vi "Phase and Amplitude Matching 2012NIVerified.vi"() -> ()   [LabVIEW 2018]
doc: "This example executes phase and/or amplitude alignment for two waveforms of the same frequency"
uses:
  <vilib>/measure/matone.llb/Extract Single Tone Information 1 Chan.vi
  <vilib>/measure/maresamp.llb/Align two Waveforms (continuous).vi
  <vilib>/measure/NI_MAPro.lvlib
  <vilib>/measure/NI_MABase.lvlib
panel:
  out "Processed Waveforms":waveform(dbl)[](graph)
  in  "Enable Phase Match?":bool=TRUE
  in  "Enable Amplitude Match?":bool=TRUE
  in  "Sampling Info A":cluster{"Fs":dbl, "#s":dbl}={"Fs"=1000.0, "#s"=1000.0}
  in  "Phase A":dbl=45.0
  in  "Amplitude A":dbl=5.0
  in  "Sampling Info B":cluster{"Fs":dbl, "#s":dbl}={"Fs"=1000.0, "#s"=1000.0}
  in  "Phase B":dbl=180.0
  in  "Amplitude B":dbl=1.0
  in  "Waveform Frequency":dbl=10.0
  out "Original Waveforms":waveform(dbl)[](graph)
  # "Overview: This example executes phase and/or amplitude alignment for two waveforms of the same frequency.\nRequirements: LabVIEW 2012 or compatible\nInstructions:\n1Run VI"
  # "Waveform A Properties"
  # "Waveform B Properties"
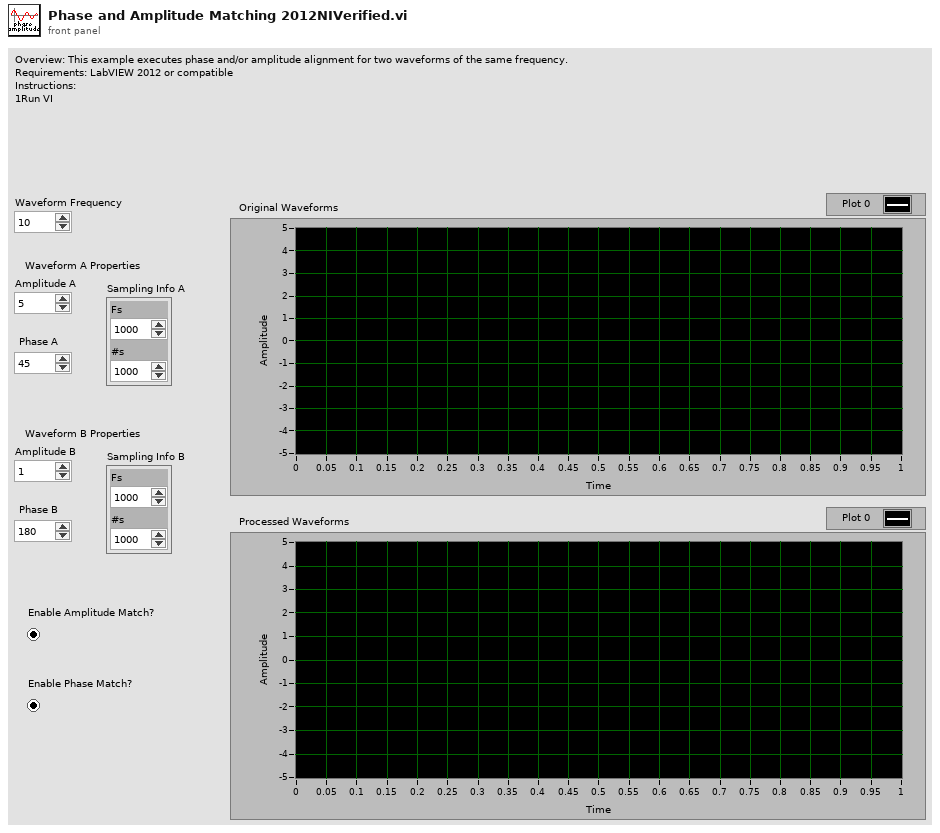
[diagram p1: front panel]
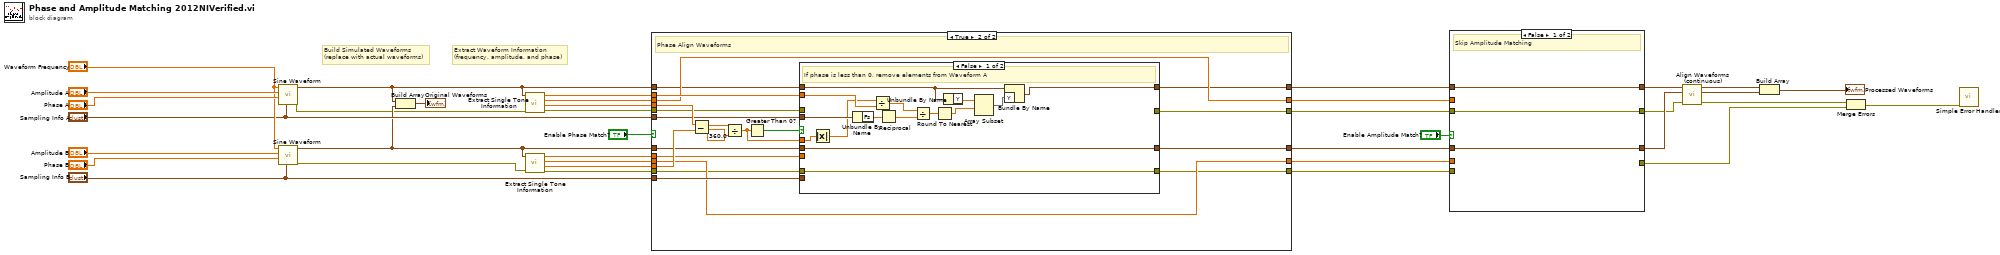
[diagram p0: block diagram]
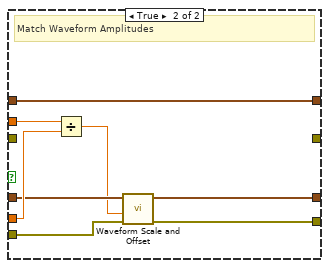
[diagram p2: hidden frame]
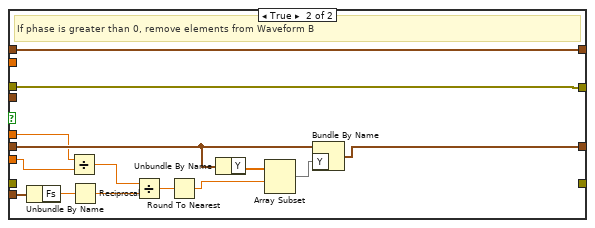
[diagram p4: hidden frame]
diagram:
  # "Extract Waveform Information\n(frequency, amplitude, and phase)"
  # "Build Simulated Waveforms\n(replace with actual waveforms)"
  n1 = call <vilib>:"Sine Waveform.vi"("sampling info"="Sampling Info A", "phase"="Phase A", "amplitude"="Amplitude A", "frequency"="Waveform Frequency") -> ("error out"=w10:errorcluster, "signal out"=w22:waveform(dbl))  [unwired: 6 in]
  n2 = call <vilib>:"Sine Waveform.vi"("sampling info"="Sampling Info B", "phase"="Phase B", "amplitude"="Amplitude B", "frequency"="Waveform Frequency") -> ("error out"=w9:errorcluster, "signal out"=w26:waveform(dbl))  [unwired: 6 in]
  n3 = Build Array(w22, w26) -> (→"Original Waveforms":waveform(dbl)[])
  n4 = call-poly <vilib>:"Extract Single Tone Information.vi"("error in (no error)"=w10, "time signal in"=w22) -> ("error out"=w6:errorcluster, "detected phase (deg)"=w27:dbl, "detected amplitude"=w28:dbl, "detected frequency"=w29:dbl)  [unwired: 4 in, 2 out]
  n5 = call-poly <vilib>:"Extract Single Tone Information.vi"("error in (no error)"=w9, "time signal in"=w26) -> ("error out"=w8:errorcluster, "detected phase (deg)"=w23:dbl, "detected amplitude"=w24:dbl, "detected frequency"=w25:dbl)  [unwired: 4 in, 2 out]
  n6 = case shown="True" "Enable Phase Match?" {
    tunnel: "Sampling Info A" -> [_ w55]
    tunnel: "Sampling Info B" -> [_ w56]
    tunnel: w22 -> [w38 w50]
    tunnel: w29 -> [_ w54]
    tunnel: w28 -> [w41 w52]
    tunnel: w27 -> [_ w61]
    tunnel: w26 -> [w39 w49]
    tunnel: w25 -> [_ w53]
    tunnel: w24 -> [w40 w51]
    tunnel: w23 -> [_ w60]
    tunnel: [w41 w52] -> w17
    tunnel: [w40 w51] -> w16
    tunnel: [w38 w47] -> w18
    tunnel: [w39 w46] -> w19
    tunnel: w8 -> [_ w45]
    tunnel: [_ w44] -> w7
    tunnel: w6 -> [_ w42]
    tunnel: [_ w43] -> w2
    frame False {
      # "Skip Phase Alignment"
    }
    frame True {
      # "Phase Align Waveforms"
      n7 = Subtract(x=w61, y=w60) -> (x-y=w59:dbl)
      n8 = Divide(x=w59, y=360.0) -> (x/y=w48:dbl)
      n9 = Greater Than 0?(x=w48) -> (x > 0?=w57:bool)
      n10 = case shown="False" w57 {
        tunnel: w56 -> [_ w90]
        tunnel: w55 -> [w71 _]
        tunnel: w54 -> [w65 _]
        tunnel: w53 -> [_ w79]
        tunnel: w50 -> [w68 w81]
        tunnel: w49 -> [w76 w85]
        tunnel: w48 -> [w64 w78]
        tunnel: [w66 w81] -> w47
        tunnel: [w76 w80] -> w46
        tunnel: w45 -> [w62 _]
        tunnel: [w62 _] -> w44
        tunnel: w42 -> [_ w77]
        tunnel: [_ w77] -> w43
        frame False {
          # "If phase is less than 0, remove elements from Waveform A"
          n11 = Absolute Value(x=w64) -> (abs(x)=w63:dbl)
          n12 = Unbundle By Name(w71) -> ("Fs"=w72:dbl)
          n13 = Divide(x=w63, y=w65) -> (x/y=w73:dbl)
          n14 = Reciprocal(x=w72) -> (1/x=w74:dbl)
          n15 = Divide(x=w73, y=w74) -> (x/y=w75:dbl)
          n16 = Round To Nearest(number=w75) -> (nearest integer value=w67:dbl)
          n17 = Unbundle By Name(w68) -> ("Y"=w69:dbl[])
          n18 = Array Subset(array=w69, index=w67) -> (w70:dbl[])  [unwired: 1 in]
          n19 = Bundle By Name(cluster=w68, "Y"=w70) -> (w66:waveform(dbl))
        }
        frame True {
          # "If phase is greater than 0, remove elements from Waveform B"
          n20 = Unbundle By Name(w90) -> ("Fs"=w89:dbl)
          n21 = Divide(x=w78, y=w79) -> (x/y=w88:dbl)
          n22 = Reciprocal(x=w89) -> (1/x=w87:dbl)
          n23 = Divide(x=w88, y=w87) -> (x/y=w83:dbl)
          n24 = Round To Nearest(number=w83) -> (nearest integer value=w82:dbl)
          n25 = Unbundle By Name(w85) -> ("Y"=w86:dbl[])
          n26 = Array Subset(array=w86, index=w82) -> (w84:dbl[])  [unwired: 1 in]
          n27 = Bundle By Name(cluster=w85, "Y"=w84) -> (w80:waveform(dbl))
        }
      }
    }
  }
  n28 = case shown="False" "Enable Amplitude Match?" {
    tunnel: w19 -> [w92 w99]
    tunnel: w18 -> [w93 w96]
    tunnel: w17 -> [_ w101]
    tunnel: w16 -> [_ w100]
    tunnel: [w93 w96] -> w15
    tunnel: [w92 w98] -> w14
    tunnel: w7 -> [_ w95]
    tunnel: [_ w94] -> w4
    tunnel: w2 -> [w91 _]
    tunnel: [w91 _] -> w1
    frame False {
      # "Skip Amplitude Matching"
    }
    frame True {
      # "Match Waveform Amplitudes"
      n29 = Divide(x=w101, y=w100) -> (x/y=w97:dbl)
      n30 = call <vilib>:"Waveform Scale and Offset.vi"("error in (no error)"=w95, "scale"=w97, "waveform in"=w99) -> ("error out"=w94:errorcluster, "waveform out"=w98:waveform(dbl))  [unwired: 7 in]
    }
  }
  n31 = call-poly <vilib>:"Align Waveforms (continuous).vi"("error in (no error)"=w1, "waveform B in"=w14, "waveform A in"=w15) -> ("error out"=w5:errorcluster, "waveform B out"=w12:waveform(dbl), "waveform A out"=w13:waveform(dbl))  [unwired: 6 in]
  n32 = Build Array(w13, w12) -> (→"Processed Waveforms":waveform(dbl)[])
  n33 = Merge Errors(w5, w4) -> (w3:errorcluster)
  n34 = call <vilib>:"Simple Error Handler.vi"("error in (no error)"=w3) -> ()  [unwired: 4 in, 5 out]
